vi "PH_Switch.set GUI elements.vi"(0 "i ref in":refnum<vi>, 5 "error in (no error)":errorcluster) -> (14 "i ref out":refnum<vi>, 19 "error out":errorcluster)   [LabVIEW 2014, in "PH_Switch.lvlib"]
doc: "Set GUI front panel elements depending on data base entries."
uses:
  PH_Switch.lvlib
  PH_Common/PH_Common.lvlib
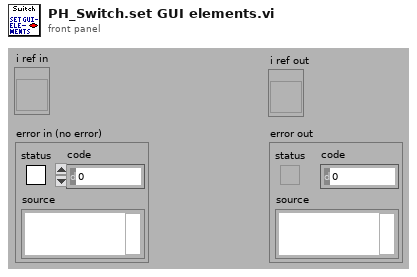
[diagram p1: front panel]
types:
  T1 = typedef "PH_Switch.lvlib/PH_Switch.i attribute.ctl" = cluster{"GUI Refs":T2, "Status true":T3, "Status false":T3, "Status Switch State":T3, "remote controlled":bool, "Tagname":cluster{"Switch":string, "True":string, "False":string}, "Beckhoff Instance":string, "Caption":cluster{"True":string, "False":string}, "Default State":string}
  T2 = typedef "PH_Switch.lvlib/PH_Switch.GUI Refs.ctl" = cluster{"true":refnum<vi>, "false":refnum<vi>, "Switch_state":refnum<vi>, "GUI-Knob":refnum<vi>, "Delete":refnum<vi>, "Function Textfield":refnum<vi>}
  T3 = typedef "PH_StatusHandler.lvlib/PH_StatusHandler.Status.ctl" = i16
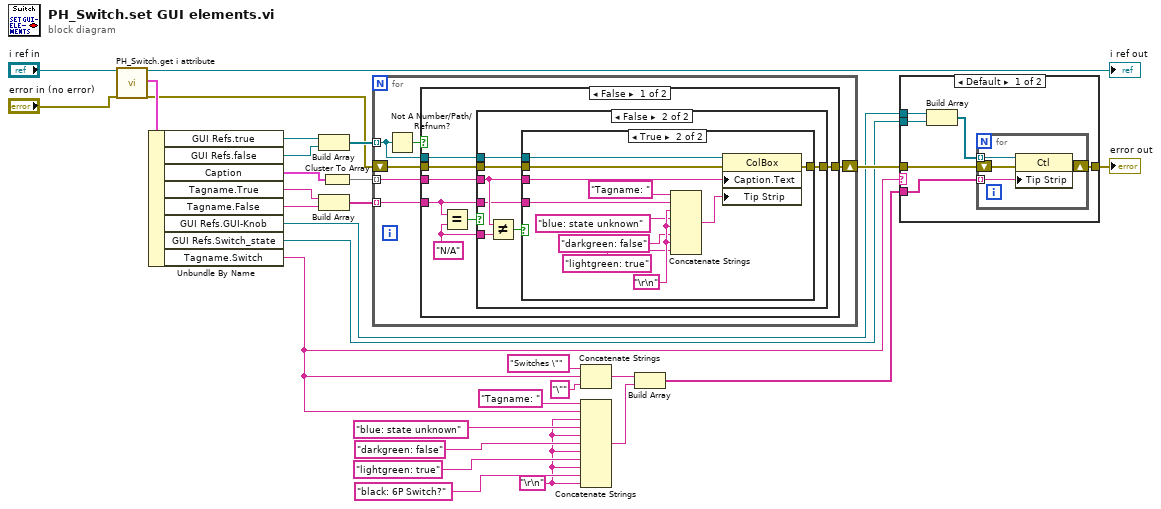
[diagram p0: block diagram]
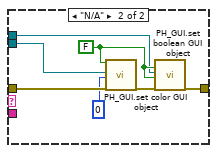
[diagram p2: hidden frame]
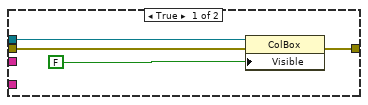
[diagram p3: hidden frame]
diagram:
  w14 = "\r\n"
  n1 = call "PH_Switch.get i attribute.vi"("i ref in"="i ref in", "error in (no error)"="error in (no error)") -> ("i ref out"=→"i ref out":refnum<vi>, "i attribute"=w29:T1, "error out"=w10:errorcluster)  [unwired: 15 in]
  n2 = Unbundle By Name(w29) -> ("GUI Refs.true"=w7:refnum<vi>, "GUI Refs.false"=w6:refnum<vi>, "Caption"=w8:cluster{"True":string, "False":string}, "Tagname.True"=w12:string, "Tagname.False"=w13:string, "GUI Refs.GUI-Knob"=w4:refnum<vi>, "GUI Refs.Switch_state"=w3:refnum<vi>, "Tagname.Switch"=w5:string)
  n3 = Build Array(w7, w6) -> (w26:refnum<vi>[])
  n4 = Build Array(w12, w13) -> (w25:string[])
  n5 = Cluster To Array(cluster=w8) -> (array=w9:string[])
  n6 = for {
    tunnel: w9 -> [w35] mode=indexing
    tunnel: w26 -> [w33] mode=indexing
    tunnel: w25 -> [w31] mode=indexing
    shift-right: [w30] -> w24
    shift-left: w10 -> [w32]
    n7 = Not A Number/Path/Refnum?(number/path/refnum=w33) -> (NaN/Path/Refnum?=w34:bool)
    n8 = case shown="False" w34 {
      tunnel: w35 -> [w42 _]
      tunnel: w31 -> [w36 _]
      tunnel: [w40 w66] -> w30
      tunnel: w32 -> [w39 w66]
      tunnel: w33 -> [w38 _]
      frame False {
        w37 = "N/A" ("x")
        n9 = Equal?(x=w36, y=w37) -> (x = y?=w41:bool)
        n10 = case shown="False" w41 {
          tunnel: w38 -> [w46 w53]
          tunnel: w39 -> [w45 w52]
          tunnel: [w44 w51] -> w40
          tunnel: w42 -> [_ w48]
          tunnel: w37 -> [_ w49]
          tunnel: w36 -> [_ w47]
          frame True {
            n11 = property class="ColBox"(reference=w46, error in=w45, "Visible"=FALSE) -> (error out=w44:errorcluster)  [unwired: 1 out]
          }
          frame False {
            n12 = Not Equal?(x=w48, y=w49) -> (x != y?=w50:bool)
            n13 = case shown="True" w50 {
              tunnel: w53 -> [_ w65]
              tunnel: w52 -> [w54 w64]
              tunnel: [w54 w63] -> w51
              tunnel: w48 -> [_ w62]
              tunnel: w47 -> [_ w56]
              frame False {
              }
              frame True {
                w60 = "\r\n"
                n14 = Concatenate Strings("Tagname: ", w56, w60, "blue: state unknown", w60, "darkgreen: false", w60, "lightgreen: true") -> (w55:string)
                n15 = property class="ColBox"(reference=w65, error in=w64, "Caption.Text"=w62, "Tip Strip"=w55) -> (error out=w63:errorcluster)  [unwired: 1 out]
              }
            }
          }
        }
      }
      frame True {
      }
    }
  }
  n16 = Concatenate Strings("Switches \"" ("string"), w5, "\"" ("string")) -> (w2:string)
  n17 = Concatenate Strings("Tagname: ", w5, w14, "blue: state unknown", w14, "darkgreen: false", w14, "lightgreen: true", w14, "black: 6P Switch?" ("string"), w14) -> (w17:string)
  n18 = Build Array(w2, w17) -> (w16:string[])
  n19 = case shown="Default" w5 {
    tunnel: [w71 w82] -> w1
    tunnel: w24 -> [w72 w81]
    tunnel: w16 -> [w70 _]
    tunnel: w4 -> [w68 w78]
    tunnel: w3 -> [w67 w77]
    frame Default {
      n20 = Build Array(w68, w67) -> (w69:refnum<vi>[])
      n21 = for {
        tunnel: w69 -> [w74] mode=indexing
        shift-right: [w75] -> w71
        shift-left: w72 -> [w76]
        tunnel: w70 -> [w73] mode=indexing
        n22 = property class="Ctl"(reference=w74, error in=w76, "Tip Strip"=w73) -> (error out=w75:errorcluster)  [unwired: 1 out]
      }
    }
    frame "N/A" {
      w80 = FALSE ("Value")
      n23 = call "PH_GUI.set color GUI object.vi"("Visible? (true)"=w80, "GUI object Ref"=w77, "State"=0, "error in (no error)"=w81) -> ("error out"=w83:errorcluster)  [unwired: 15 in]
      n24 = call "PH_GUI.set boolean GUI object.vi"("Visible (true)"=w80, "Boolean Knob GUI Ref"=w78, "Value"=w80, "error in (no error)"=w83) -> ("error out"=w82:errorcluster)  [unwired: 15 in]
    }
  }
  "error out" <- w1
